vi "Update messages.vi"(1 "Message to add":string, 2 "Old message string":string) -> (0 "New message string":string)   [LabVIEW 2014]
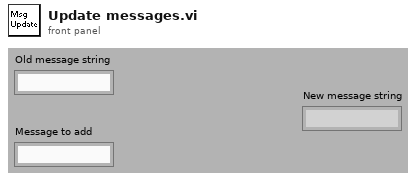
[diagram p1: front panel]
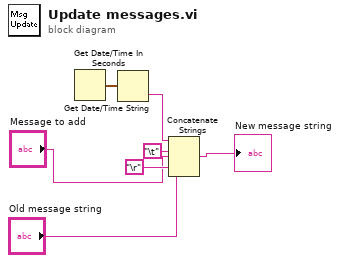
[diagram p0: block diagram]
diagram:
  n1 = Get Date/Time In Seconds() -> (seconds since 1Jan1904=w6:timestamp)
  n2 = Get Date/Time String(seconds (now)=w6) -> (time string=w4:string)  [unwired: 3 out]
  n3 = Concatenate Strings(w4, "\t" ("string"), "Message to add", "\r", "Old message string") -> (→"New message string":string)
